vi "Retrieve Frame And Script Scratch VI.vi"(8 "error in":errorcluster, 11 "FlatSeqFrame Refnum":refnum<vi>) -> (0 "error out":errorcluster, 2 "scratch VI":refnum<vi>, 3 "FlatSeqFrame Refnum (out)":refnum<vi>)   [LabVIEW 2009]
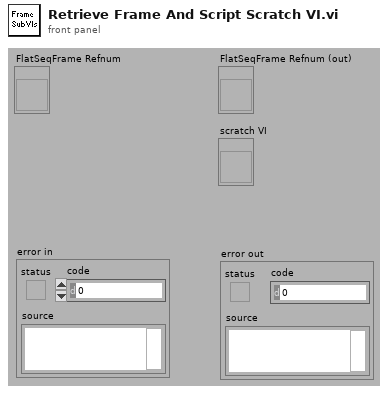
[diagram p1: front panel]
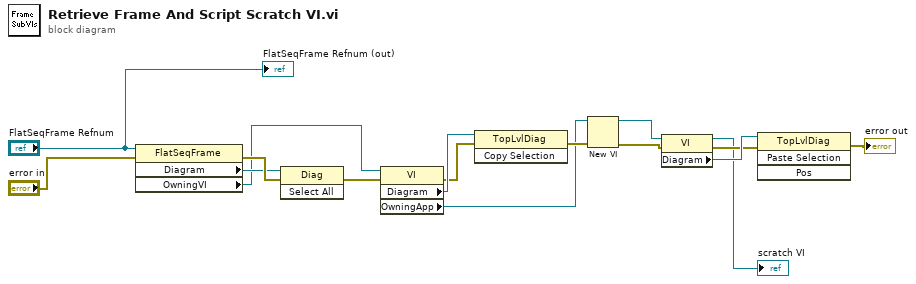
[diagram p0: block diagram]
diagram:
  n1 = property class="FlatSeqFrame"(reference="FlatSeqFrame Refnum", error in="error in") -> (error out=w9:errorcluster, "Diagram"=w8:refnum<vi>, "OwningVI"=w3:refnum<vi>)  [unwired: 1 out]
  n2 = invoke class="Diag" method="Select All"(reference=w8, error in=w9) -> (error out=w7:errorcluster)  [unwired: 1 in, 2 out]
  n3 = property class="VI"(reference=w3, error in=w7) -> (error out=w11:errorcluster, "Diagram"=w12:refnum<vi>, "OwningApp"=w6:refnum<vi>)  [unwired: 1 out]
  n4 = invoke class="TopLvlDiag" method="Copy Selection"(reference=w12, error in=w11) -> (error out=w16:errorcluster)  [unwired: 1 in, 2 out]
  n5 = New VI(8:w16, 11:w6) -> (0:w15:errorcluster, 3:w10:refnum<vi>)  [unwired: 5 in]
  n6 = property class="VI"(reference=w10, error in=w15) -> (reference out=→"scratch VI":refnum<vi>, error out=w13:errorcluster, "Diagram"=w14:refnum<vi>)
  n7 = invoke class="TopLvlDiag" method="Paste Selection"(reference=w14, error in=w13) -> (error out=→"error out":errorcluster)  [unwired: 2 in, 3 out]
  "FlatSeqFrame Refnum (out)" <- "FlatSeqFrame Refnum"
